vi "Make Y=0 waveform.vi"(1 "signal out 2":waveform(dbl)) -> (0 "signal out":waveform(dbl))   [LabVIEW 2018, in "Waveform Control.xctl"]
doc: "Generates a waveform that is all 0, but with same time information as the input array and returns both as an array of waveforms. Used to generate the plots for the graphical waveform display"
uses:
  Waveform Control.xctl
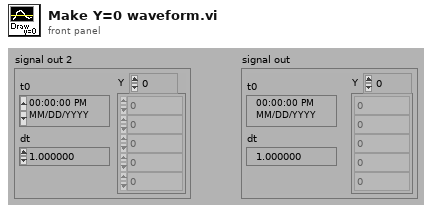
[diagram p1: front panel]
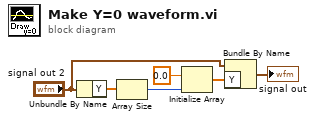
[diagram p0: block diagram]
diagram:
  n1 = Unbundle By Name("signal out 2") -> ("Y"=w1:dbl[])
  n2 = Array Size(array=w1) -> (size(s)=w2:i32)
  n3 = Initialize Array(0.0 ("element"), w2) -> (w5:dbl[])
  n4 = Bundle By Name(cluster="signal out 2", "Y"=w5) -> (→"signal out":waveform(dbl))
